vi "Valve Tag Names.vi"(11 "Process Name":string) -> (3 "Valve Tags":T1, 4 "All Boolean Tags":string[](array[string]), 5 "All  Numeric Tags":string[](array[string]))   [LabVIEW 2018, in "VICI Electronic Actuator.lvlib"]
uses:
  D-O Module Folder/DIO Valve/VICI Electronic Actuator.lvlib
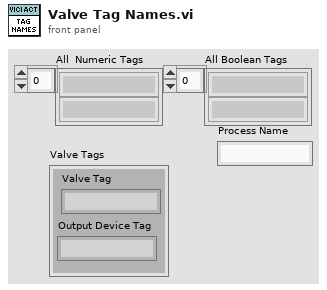
[diagram p1: front panel]
types:
  T1 = cluster{"Valve Tag":string, "Output Device Tag":string}
  T2 = cluster{"Valve Value":string, "Valve Error":string}
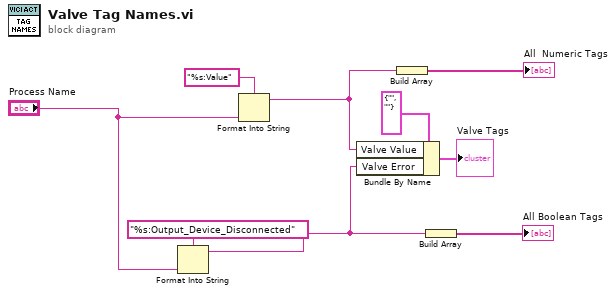
[diagram p0: block diagram]
diagram:
  n1 = Format Into String(format string="%s:Output_Device_Disconnected", "Process Name") -> (resulting string=w1:string)  [unwired: 2 in, 1 out]
  n2 = Format Into String(format string="%s:Value", "Process Name") -> (resulting string=w3:string)  [unwired: 2 in, 1 out]
  n3 = Bundle By Name(cluster=T2 {"Valve Value"="", "Valve Error"=""} ("Scale Tags 2"), "Valve Value"=w3, "Valve Error"=w1) -> (→"Valve Tags":T2)
  n4 = Build Array(w3) -> (→"All  Numeric Tags":string[])
  n5 = Build Array(w1) -> (→"All Boolean Tags":string[])
